vi "SSP - set value BOOL.vi"(8 "error in (no error)":errorcluster, 11 "JSON string":string) -> (0 "error out":errorcluster, 3 "value":string)   [LabVIEW 2020, in "ui-testing.lvlib"]
doc: "copyright: Thomas Zilliox©"
uses:
  ui-testing.lvlib
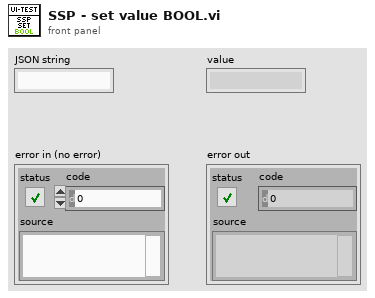
[diagram p1: front panel]
types:
  T1 = cluster{"control":string, "subpanel":string, "subsubpanel":string, "value":bool}
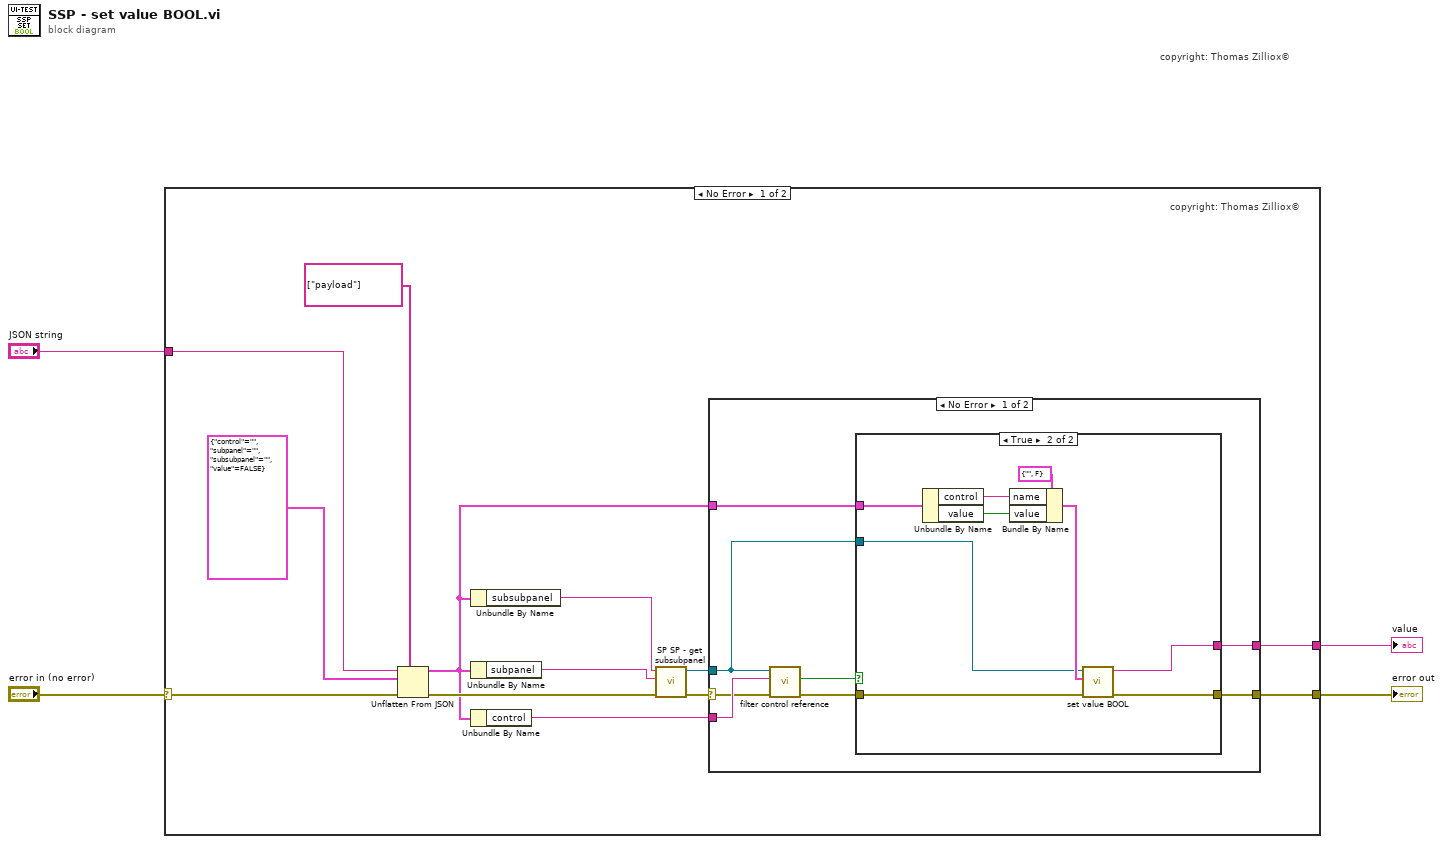
[diagram p0: block diagram]
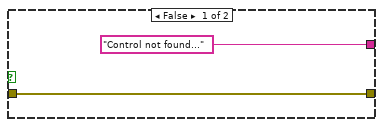
[diagram p2: hidden frame]
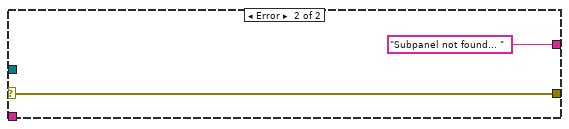
[diagram p3: hidden frame]
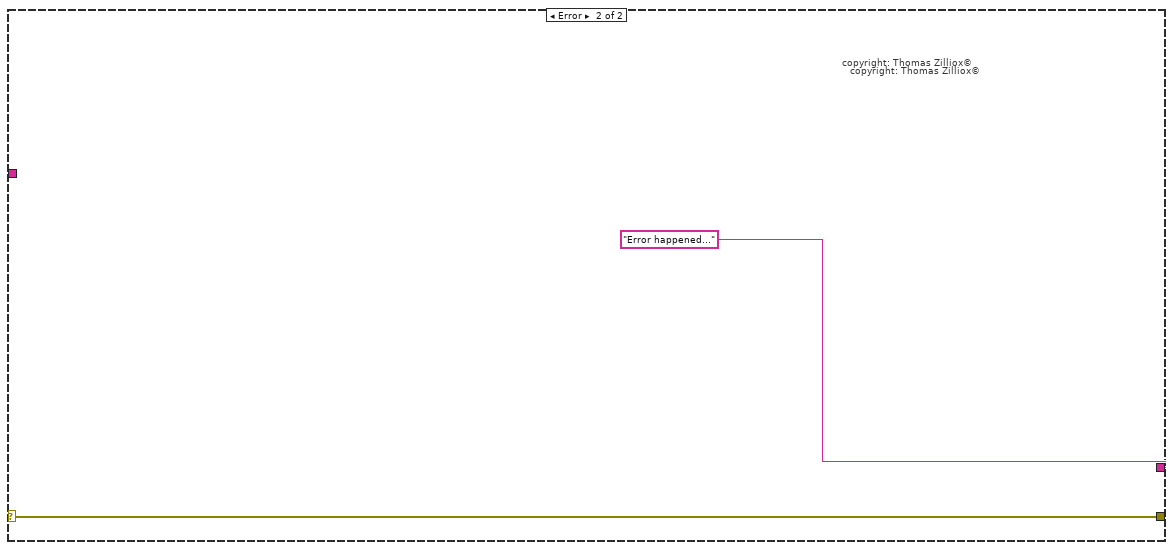
[diagram p4: hidden frame]
diagram:
  # "copyright: Thomas Zilliox©"
  n1 = case shown="No Error" "error in (no error)" {
    selector: "error in (no error)" -> [w13 w40]
    tunnel: "JSON string" -> [w15 _]
    tunnel: [w14 w40] -> w3
    tunnel: [w12 "Error happened..."] -> w1
    frame No Error {
      # "copyright: Thomas Zilliox©"
      n2 = Unflatten From JSON(path=string[] ["payload"], JSON string=w15, type and defaults=T1 {"control"="", "subpanel"="", "subsubpanel"="", "value"=FALSE}, error in (no error)=w13) -> (value=w9:T1, error out=w16:errorcluster)  [unwired: 3 in]
      n3 = Unbundle By Name(w9) -> ("subsubpanel"=w8:string)
      n4 = Unbundle By Name(w9) -> ("subpanel"=w7:string)
      n5 = Unbundle By Name(w9) -> ("control"=w10:string)
      n6 = call "SP SP - get subsubpanel.vi"("error in (no error)"=w16, "subpanel"=w7, "subsubpanel"=w8) -> ("error out"=w5:errorcluster, "SubSubPanel VI"=w6:refnum<vi>)  [unwired: 5 in, 2 out]
      n7 = case shown="No Error" w5 {
        selector: w5 -> [w20 w37]
        tunnel: [w25 w37] -> w14
        tunnel: w6 -> [w22 _]
        tunnel: w10 -> [w21 _]
        tunnel: [w24 "Subpanel not found... " ("result string")] -> w12
        tunnel: w9 -> [w23 _]
        frame No Error {
          n8 = call "filter control reference.vi"("error in (no error)"=w20, "Control label"=w21, "VI (Caller)"=w22) -> ("error out"=w18:errorcluster, "Control found"=w19:bool)  [unwired: 6 in, 1 out]
          n9 = case shown="True" w19 {
            tunnel: w18 -> [w27 w30]
            tunnel: [w27 w28] -> w25
            tunnel: ["Control not found..." ("result string") w29] -> w24
            tunnel: w23 -> [_ w32]
            tunnel: w22 -> [_ w31]
            frame False {
            }
            frame True {
              n10 = Unbundle By Name(w32) -> ("control"=w33:string, "value"=w34:bool)
              n11 = Bundle By Name(cluster=cluster{"name":string, "value":bool} {"name"="", "value"=FALSE} ("Payload"), "name"=w33, "value"=w34) -> (w35:cluster{"name":string, "value":bool})
              n12 = call "set value BOOL.vi"("error in (no error)"=w30, "Payload"=w35, "VI Ref"=w31) -> ("error out"=w28:errorcluster, "return value"=w29:string)  [unwired: 7 in]
            }
          }
        }
        frame Error {
        }
      }
    }
    frame Error {
      # "copyright: Thomas Zilliox©"
      # "copyright: Thomas Zilliox©"
    }
  }
  "error out" <- w3
  "value" <- w1
